vi "Nand3 15.vi"(1 "C":bool, 2 "B":bool, 3 "A":bool) -> (0 "Boolean":bool)   [LabVIEW 2018]
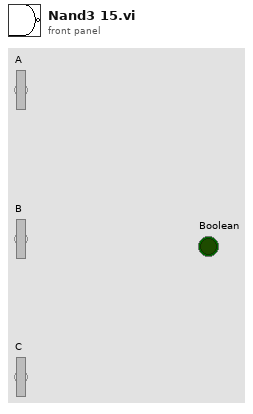
[diagram p1: front panel]
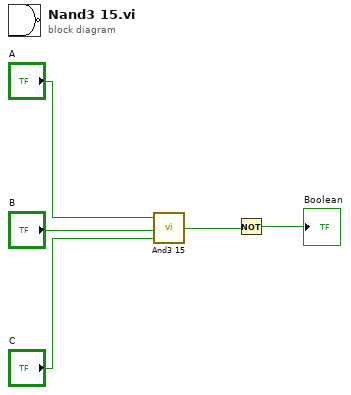
[diagram p0: block diagram]
diagram:
  n1 = call "And3 15.vi"("C"="C", "B"="B", "A"="A") -> ("out"=w2:bool)
  n2 = Not(x=w2) -> (.not. x?=→"Boolean":bool)
